vi "Find Parse State Queue from Case Structure.vi"(8 "error in (no error)":errorcluster, 11 "CaseStructure":refnum<vi>) -> (0 "error out":errorcluster, 1 "CaseStructure":refnum<vi>, 2 "Parse State Queue":refnum<vi>)   [LabVIEW 2017, in "CSM-Helper.lvclass"]
uses:
  CSM-Helper.lvclass
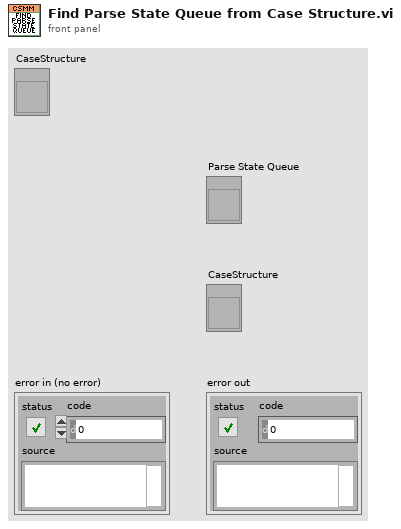
[diagram p1: front panel]
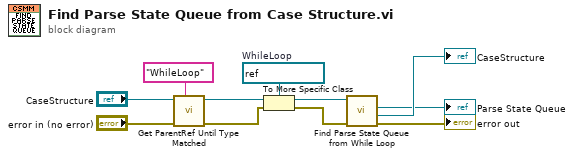
[diagram p0: block diagram]
diagram:
  w8 = refnum<vi> refnum  # WhileLoop
  n1 = call "Get ParentRef Until Type Matched.vi"("Class Name"="WhileLoop", "Error in"="error in (no error)", "reference in"="CaseStructure") -> ("Error out"=w6:errorcluster, "Target Ref"=w10:refnum<vi>)  [unwired: 5 in]
  n2 = To More Specific Class(target class=w8, reference=w10, error in=w6) -> (specific class reference=w9:refnum<vi>, error out=w7:errorcluster)
  n3 = call "Find Parse State Queue from While Loop.vi"("error in (no error)"=w7, "WhileLoop in"=w9) -> ("error out"=→"error out":errorcluster, "CaseStructure"=→"CaseStructure":refnum<vi>, "Parse State Queue"=→"Parse State Queue":refnum<vi>)  [unwired: 6 in, 1 out]
